vi "Merge Array Sizes.vi"(2 "Sizes 2":i32[](array[numeric]), 3 "Sizes":i32[](array[numeric])) -> (1 "Sizes out":i32[](array[numeric]))   [LabVIEW 2013, in "JKI JSON Serialization.lvlib" / "JSON Deserializer.lvclass"]
uses:
  JSON Deserializer.lvclass
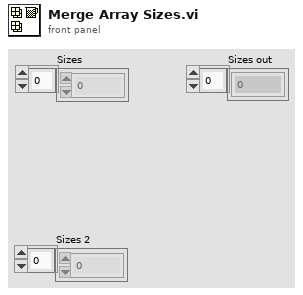
[diagram p1: front panel]
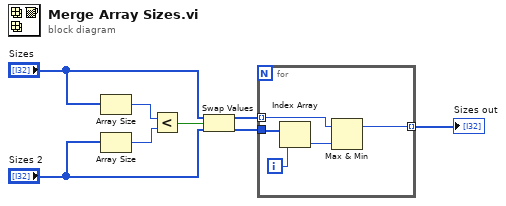
[diagram p0: block diagram]
diagram:
  n1 = Array Size(array="Sizes") -> (size(s)=w8:i32)
  n2 = Array Size(array="Sizes 2") -> (size(s)=w7:i32)
  n3 = Less?(x=w8, y=w7) -> (x < y?=w6:bool)
  n4 = Swap Values(12:"Sizes", 13:w6, 14:"Sizes 2") -> (1:w2:i32[], 3:w3:i32[])
  n5 = for {
    tunnel: w3 -> [w13]
    tunnel: w2 -> [w10] mode=indexing
    tunnel: [w9] -> w1 mode=indexing
    i -> [w12]
    n6 = Index Array(array=w13, index=w12) -> (element=w11:i32)
    n7 = Max & Min(x=w10, y=w11) -> (max(x,y)=w9:i32)  [unwired: 1 out]
  }
  "Sizes out" <- w1
